vi "S2DS_ConditionForWriteToBufferNew.vi"(3 "Measurement":bool, 6 "Scan parameters in":T1 {"Y data taking" items=["in both direction", "in up direction only", "in down direction only"]; "X data taking" items=["in both direction", "in up direction only", "in down direction only"]}) -> (1 "Update on?":bool, 2 "Measurement on?":bool)   [LabVIEW 2025]
uses:
  TYPE DEFS/S2DS_Sweep Info.ctl
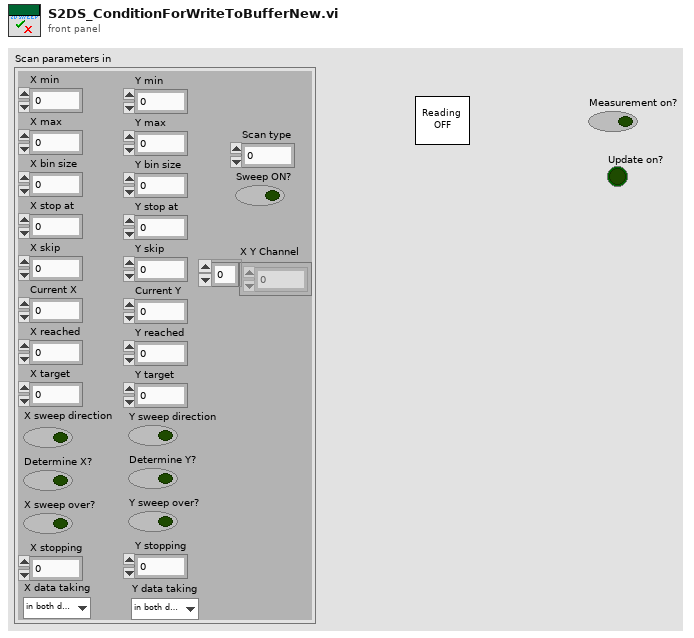
[diagram p1: front panel]
types:
  T1 = typedef "S2DS_Sweep Info.ctl" = cluster{"X min":ext, "X max":dbl, "Y min":dbl, "Y max":dbl, "X bin size":dbl, "Y bin size":dbl, "X stop at":dbl, "Y stop at":dbl, "X skip":u64, "Y skip":u64, "Current X":dbl, "Current Y":dbl, "X reached":i32, "Y reached":i32, "X target":dbl, "Y target":dbl, "Sweep ON?":bool, "X sweep direction":bool, "Y sweep direction":bool, "Determine X?":bool, "Determine Y?":bool, "X sweep over?":bool, "Y sweep over?":bool, "Scan type":i32, "X stopping":i32, "Y stopping":i32, "X Y Channel":u16[], "X data taking":u16, "Y data taking":u16}
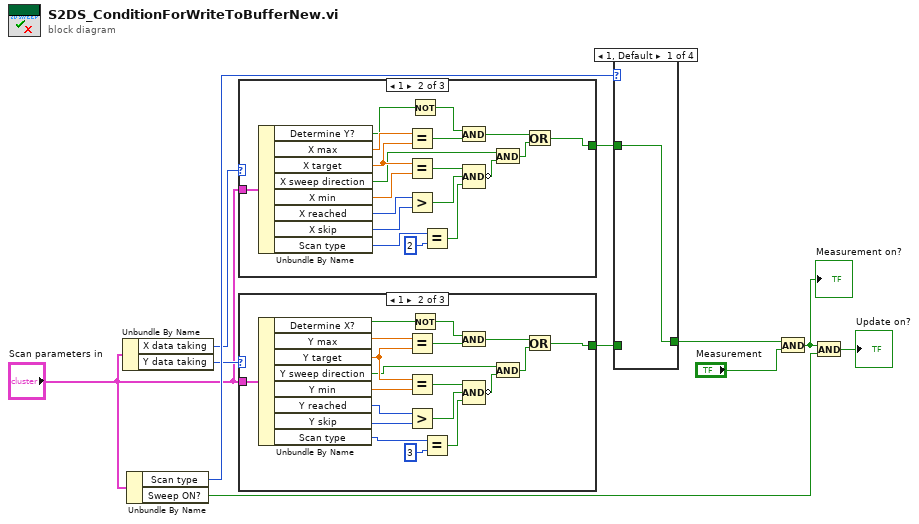
[diagram p0: block diagram]
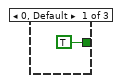
[diagram p2: hidden frame]
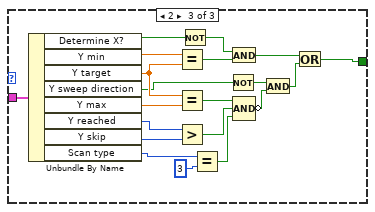
[diagram p3: hidden frame]
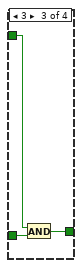
[diagram p5: hidden frame]
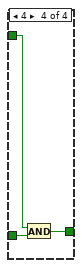
[diagram p6: hidden frame]
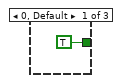
[diagram p7: hidden frame]
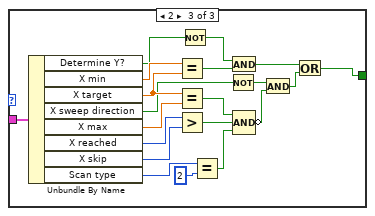
[diagram p8: hidden frame]
diagram:
  n1 = Unbundle By Name("Scan parameters in") -> ("X data taking"=w4:u16, "Y data taking"=w3:u16)
  n2 = Unbundle By Name("Scan parameters in") -> ("Scan type"=w10:i32, "Sweep ON?"=w7:bool)
  n3 = case shown="1" w4 {
    tunnel: [TRUE w29 w49] -> w11
    tunnel: "Scan parameters in" -> [_ w30 w50]
    frame 0, Default {
    }
    frame 1 {
      n4 = Unbundle By Name(w30) -> ("Determine Y?"=w26:bool, "X max"=w31:dbl, "X target"=w24:dbl, "X sweep direction"=w17:bool, "X min"=w23:ext, "X reached"=w22:i32, "X skip"=w21:u64, "Scan type"=w15:i32)
      n5 = Equal?(x=w31, y=w24) -> (x = y?=w28:bool)
      n6 = Equal?(x=w24, y=w23) -> (x = y?=w20:bool)
      n7 = Greater?(x=w22, y=w21) -> (0:w19:bool)
      n8 = Not(x=w26) -> (.not. x?=w25:bool)
      n9 = Equal?(x=w15, y=2) -> (x = y?=w13:bool)
      n10 = And(x=w25, y=w28) -> (x .and. y?=w27:bool)
      n11 = Compound Arithmetic op=AND(w20, w19, w13) -> (invert w18:bool)
      n12 = And(x=w17, y=w18) -> (x .and. y?=w16:bool)
      n13 = Or(x=w27, y=w16) -> (x .or. y?=w29:bool)
    }
    frame 2 {
      n14 = Unbundle By Name(w50) -> ("Determine Y?"=w46:bool, "X min"=w51:ext, "X target"=w44:dbl, "X sweep direction"=w33:bool, "X max"=w43:dbl, "X reached"=w42:i32, "X skip"=w41:u64, "Scan type"=w36:i32)
      n15 = Equal?(x=w51, y=w44) -> (x = y?=w48:bool)
      n16 = Equal?(x=w44, y=w43) -> (x = y?=w40:bool)
      n17 = Greater?(x=w42, y=w41) -> (0:w39:bool)
      n18 = Not(x=w46) -> (.not. x?=w45:bool)
      n19 = Equal?(x=w36, y=2) -> (x = y?=w34:bool)
      n20 = Not(x=w33) -> (.not. x?=w32:bool)
      n21 = And(x=w45, y=w48) -> (x .and. y?=w47:bool)
      n22 = Compound Arithmetic op=AND(w40, w39, w34) -> (invert w38:bool)
      n23 = And(x=w32, y=w38) -> (x .and. y?=w37:bool)
      n24 = Or(x=w47, y=w37) -> (x .or. y?=w49:bool)
    }
  }
  n25 = case shown="1" w3 {
    tunnel: [TRUE w69 w89] -> w1
    tunnel: "Scan parameters in" -> [_ w70 w90]
    frame 0, Default {
    }
    frame 1 {
      n26 = Unbundle By Name(w70) -> ("Determine X?"=w66:bool, "Y max"=w71:dbl, "Y target"=w64:dbl, "Y sweep direction"=w57:bool, "Y min"=w63:dbl, "Y reached"=w62:i32, "Y skip"=w61:u64, "Scan type"=w55:i32)
      n27 = Equal?(x=w71, y=w64) -> (x = y?=w68:bool)
      n28 = Equal?(x=w64, y=w63) -> (x = y?=w60:bool)
      n29 = Greater?(x=w62, y=w61) -> (0:w59:bool)
      n30 = Not(x=w66) -> (.not. x?=w65:bool)
      n31 = Equal?(x=w55, y=3) -> (x = y?=w53:bool)
      n32 = And(x=w65, y=w68) -> (x .and. y?=w67:bool)
      n33 = Compound Arithmetic op=AND(w60, w59, w53) -> (invert w58:bool)
      n34 = And(x=w57, y=w58) -> (x .and. y?=w56:bool)
      n35 = Or(x=w67, y=w56) -> (x .or. y?=w69:bool)
    }
    frame 2 {
      n36 = Unbundle By Name(w90) -> ("Determine X?"=w86:bool, "Y min"=w91:dbl, "Y target"=w84:dbl, "Y sweep direction"=w73:bool, "Y max"=w83:dbl, "Y reached"=w82:i32, "Y skip"=w81:u64, "Scan type"=w76:i32)
      n37 = Equal?(x=w91, y=w84) -> (x = y?=w88:bool)
      n38 = Equal?(x=w84, y=w83) -> (x = y?=w80:bool)
      n39 = Greater?(x=w82, y=w81) -> (0:w79:bool)
      n40 = Not(x=w86) -> (.not. x?=w85:bool)
      n41 = Equal?(x=w76, y=3) -> (x = y?=w74:bool)
      n42 = Not(x=w73) -> (.not. x?=w72:bool)
      n43 = And(x=w85, y=w88) -> (x .and. y?=w87:bool)
      n44 = Compound Arithmetic op=AND(w80, w79, w74) -> (invert w78:bool)
      n45 = And(x=w72, y=w78) -> (x .and. y?=w77:bool)
      n46 = Or(x=w87, y=w77) -> (x .or. y?=w89:bool)
    }
  }
  n47 = case shown="1, Default" w10 {
    tunnel: [w92 w93 w94 w97] -> w8
    tunnel: w11 -> [w92 _ w96 w99]
    tunnel: w1 -> [_ w93 w95 w98]
    frame 1, Default {
    }
    frame 2 {
    }
    frame 3 {
      n48 = And(x=w96, y=w95) -> (x .and. y?=w94:bool)
    }
    frame 4 {
      n49 = And(x=w99, y=w98) -> (x .and. y?=w97:bool)
    }
  }
  n50 = And(x=w8, y="Measurement") -> (x .and. y?=w6:bool)
  "Measurement on?" <- w6
  n51 = And(x=w6, y=w7) -> (x .and. y?=→"Update on?":bool)
